vi "NISE.remote.Property Node Read Core.vi"(8 "error in (no error)":errorcluster, 10 "property":string, 11 "SLSC Remote in":refnum<class "SLSC Interface.lvclass">) -> (0 "error out":errorcluster, 2 "JSON Value out":refnum<class "JSON Value.lvclass">, 3 "SLSC Remote out":refnum<class "SLSC Interface.lvclass">)   [LabVIEW 2016, in "SLSC Interface.lvclass"]
uses:
  SLSC Interface Class/SLSC Interface.lvclass
  <vilib>/NI/JSON Support for LabVIEW/JSON Value/JSON Value.lvclass
  SLSC Interface Class/SLSC Interface.lvclass/SLSC Interface.ctl
  SLSC Interface Class/NISE.Read client handle.vi
  SLSC Interface Class/NISE.Read URL.vi
  SLSC Interface Class/NISE.Read session.vi
  <vilib>/NI/NI JSONRPC Server Framework/Classes/Server/server.Format Client Request (Auto-Increment).vi
  <vilib>/httpClient/POSTBuffer.vi
  <vilib>/httpClient/LabVIEWHTTPClient.lvlib
  <vilib>/NI/NI JSONRPC Server Framework/Classes/Server/JSONRPC Server.lvclass
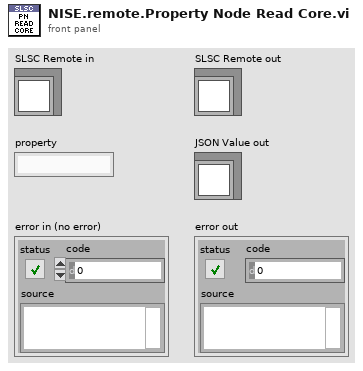
[diagram p1: front panel]
types:
  T1 = typedef "LabVIEWHTTPClient.lvlib/ClientHandle.ctl" = refnum<k1>
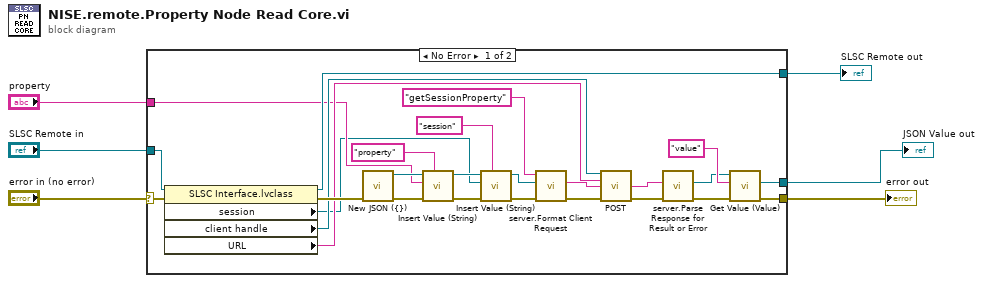
[diagram p0: block diagram]
diagram:
  n1 = case shown="No Error" "error in (no error)" {
    selector: "error in (no error)" -> [w30 w33]
    tunnel: "SLSC Remote in" -> [w32 w34]
    tunnel: [w31 w34] -> w3
    tunnel: [w15 w33] -> w4
    tunnel: [w16 _] -> w1
    tunnel: "property" -> [w9 _]
    frame No Error {
      n2 = property class="SLSC Interface.lvclass"(reference=w32, error in=w30) -> (reference out=w31:refnum<class "SLSC Interface.lvclass">, error out=w29:errorcluster, "session"=w8:refnum<k21>, "client handle"=w22:T1, "URL"=w21:string)
      n3 = call <vilib>:"New JSON ({}).vi"("error in (no error)"=w29) -> ("error out"=w28:errorcluster, "JSON Value out"=w12:refnum<class "JSON Value.lvclass">)  [unwired: 9 in]
      n4 = call <vilib>:"Insert Value (String).vi"("key"="property" ("Name"), "error in (no error)"=w28, "value"=w9, "JSON Value in"=w12) -> ("error out"=w25:errorcluster, "JSON Value out"=w11:refnum<class "JSON Value.lvclass">)  [unwired: 5 in, 1 out]
      n5 = call <vilib>:"Insert Value (String).vi"("key"="session" ("Name"), "error in (no error)"=w25, "value"=w8, "JSON Value in"=w11) -> ("error out"=w23:errorcluster, "JSON Value out"=w24:refnum<class "JSON Value.lvclass">)  [unwired: 5 in, 1 out]
      n6 = call-poly <vilib>:"server.Format Client Request.vi"("error in (no error)"=w23, "JSON Value in"=w24, "method"="getSessionProperty") -> ("error out"=w20:errorcluster, "Request String"=w26:string)  [unwired: 7 in]
      n7 = call-poly <vilib>:"POST.vi"("client handle"=w22, "url"=w21, "buffer"=w26, "error in (no error)"=w20) -> ("body"=w19:string, "error out"=w18:errorcluster)  [unwired: 8 in, 2 out]
      n8 = call <vilib>:"server.Parse Response for Result or Error.vi"("error in"=w18, "Response String In"=w19) -> ("error out"=w10:errorcluster, "JSON Value out"=w7:refnum<class "JSON Value.lvclass">)  [unwired: 7 in, 1 out]
      n9 = call <vilib>:"Get Value (Value).vi"("error in (no error)"=w10, "key"="value" ("Parameter Name"), "JSON Value in"=w7) -> ("error out"=w15:errorcluster, "JSON Value out"=w16:refnum<class "JSON Value.lvclass">)  [unwired: 7 in]
    }
    frame Error {
    }
  }
  "error out" <- w4
  "SLSC Remote out" <- w3
  "JSON Value out" <- w1
